vi "Update_buy_values.vi"(6 "MXN?":bool, 7 "Producto":string, 8 "error in (no error)":errorcluster, 9 "Cantidad":dbl, 10 "Precio":dbl, 11 "UI Actor in":refnum<class "UI Actor.lvclass">) -> (0 "error out":errorcluster, 3 "UI Actor out":refnum<class "UI Actor.lvclass">)   [LabVIEW 2019, in "UI Actor.lvlib" / "UI Actor.lvclass"]
uses:
  UI Actor.lvclass
  C:/Program Files/National Instruments/LabVIEW 2019/vi.lib/ActorFramework/Actor/Actor.lvclass
  UI Actor.lvclass/UI Actor.ctl
  <vilib>/ActorFramework/Actor/Actor.lvclass/Actor.ctl
  UI Actor Messages/Update Credit Msg/Update Credit Msg.lvclass/Update Credit Msg.ctl
  <vilib>/ActorFramework/Message Enqueuer/Message Enqueuer.lvclass/Message Enqueuer.ctl
  Actor_USD Messages/New Credit Msg/New Credit Msg.lvclass/New Credit Msg.ctl
  Actor_C_MXN Messages/Nuevo_credito Msg/Nuevo_credito Msg.lvclass/Nuevo_credito Msg.ctl
  Mensajes Messages/Update Message event Msg/Update Message event Msg.lvclass/Update Message event Msg.ctl
  <vilib>/ActorFramework/Message Enqueuer/Enqueue.vi
  UI Actor Messages/Update Credit Msg/Update Credit Msg.lvclass
  C:/Program Files/National Instruments/LabVIEW 2019/vi.lib/ActorFramework/Message/Message.lvclass
  Actor_USD Messages/New Credit Msg/New Credit Msg.lvclass
  Actor_C_MXN Messages/Nuevo_credito Msg/Nuevo_credito Msg.lvclass
  Mensajes Messages/Update Message event Msg/Update Message event Msg.lvclass
  <vilib>/ActorFramework/Message Priority Queue/Priority Enqueue.vi
  <vilib>/ActorFramework/Actor/Actor.lvclass
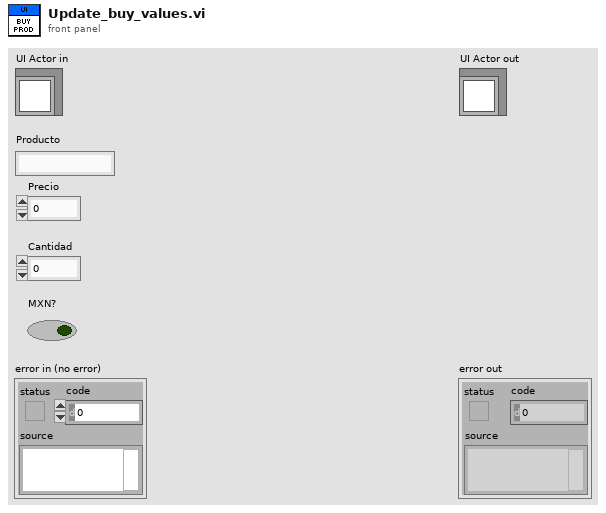
[diagram p1: front panel]
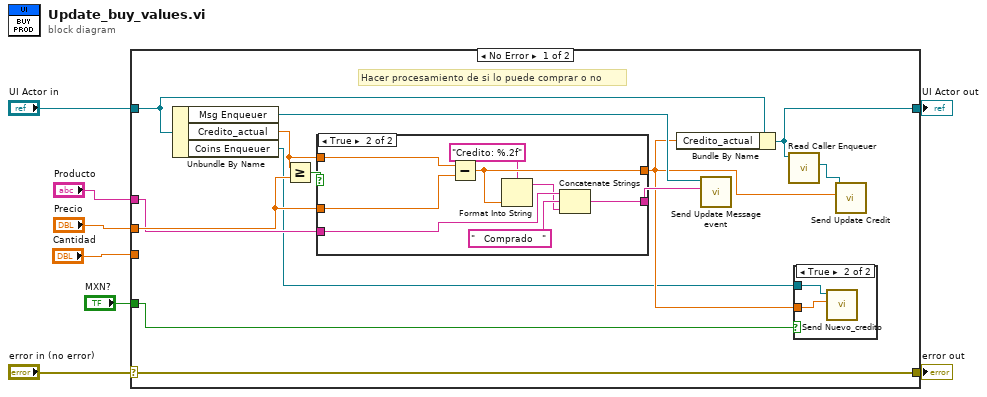
[diagram p0: block diagram]
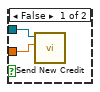
[diagram p2: hidden frame]
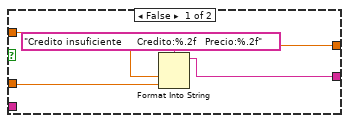
[diagram p3: hidden frame]
diagram:
  n1 = case shown="No Error" "error in (no error)" {
    selector: "error in (no error)" -> [w21 w39]
    tunnel: [w21 w39] -> w7
    tunnel: [w12 w38] -> w5
    tunnel: "UI Actor in" -> [w17 w38]
    tunnel: "Producto" -> [w16 _]
    tunnel: "Precio" -> [w18 _]
    tunnel: "Cantidad" -> [_ _]
    tunnel: "MXN?" -> [w9 _]
    frame No Error {
      # "Hacer procesamiento de si lo puede comprar o no"
      n2 = Unbundle By Name(w17) -> ("Msg Enqueuer"=w14:refnum<class "Message Enqueuer.lvclass">, "Credito_actual"=w19:dbl, "Coins Enqueuer"=w10:refnum<class "Message Enqueuer.lvclass">)
      n3 = Greater Or Equal?(x=w19, y=w18) -> (x >= y?=w20:bool)
      n4 = case shown="True" w20 {
        tunnel: w19 -> [w29 w37]
        tunnel: w18 -> [w28 w36]
        tunnel: [w29 w35] -> w11
        tunnel: w16 -> [_ w33]
        tunnel: [w26 w30] -> w15
        frame False {
          n5 = Format Into String(format string="Credito insuficiente     Credito:%.2f   Precio:%.2f", w29, w28) -> (resulting string=w26:string)  [unwired: 2 in, 1 out]
        }
        frame True {
          n6 = Subtract(x=w37, y=w36) -> (x-y=w35:dbl)
          n7 = Format Into String(format string="Credito: %.2f", w35) -> (resulting string=w31:string)  [unwired: 2 in, 1 out]
          n8 = Concatenate Strings(w33, "   Comprado   " ("string"), w31) -> (w30:string)
        }
      }
      n9 = Bundle By Name(cluster=w17, "Credito_actual"=w11) -> (w12:refnum<class "UI Actor.lvclass">)
      n10 = call "Send Update Message event.vi"("Update Msg"=w15, "Message Enqueuer"=w14) -> ()  [unwired: 8 in, 2 out]
      n11 = call <vilib>:"Read Caller Enqueuer.vi"("Actor"=w12) -> ("Caller Enqueuer"=w13:refnum<class "Message Enqueuer.lvclass">)  [unwired: 10 in]
      n12 = case shown="True" w9 {
        tunnel: w11 -> [w22 w25]
        tunnel: w10 -> [w23 w24]
        frame False {
          n13 = call "Send New Credit.vi"("Nw Credit"=w22, "Message Enqueuer"=w23) -> ()  [unwired: 8 in, 2 out]
        }
        frame True {
          n14 = call "Send Nuevo_credito.vi"("Nuevo Credito"=w25, "Message Enqueuer"=w24) -> ()  [unwired: 8 in, 2 out]
        }
      }
      n15 = call "Send Update Credit.vi"("Credito"=w11, "Message Enqueuer"=w13) -> ()  [unwired: 8 in, 2 out]
    }
    frame Error {
    }
  }
  "error out" <- w7
  "UI Actor out" <- w5
